vi "aft_FXP_LMS_Address_Generator.vi"(7 "filter length":i32, 10 "initialize x read address":u32, 11 "index":i32) -> (0 "x read address":u32, 1 "coefficient read address":u32, 2 "coefficient write enable":bool, 3 "coefficient write address":u32)   [LabVIEW 2017]
doc: "This VI generates addresses for reading and writing RAM."
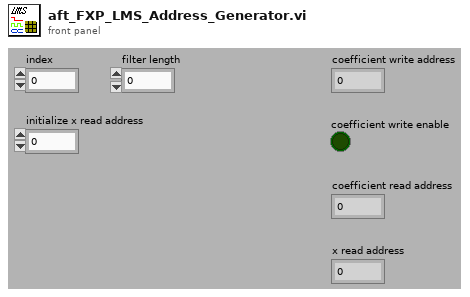
[diagram p1: front panel]
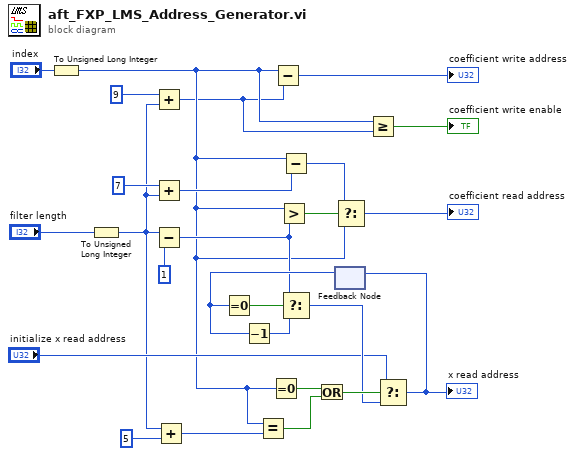
[diagram p0: block diagram]
diagram:
  n1 = To Unsigned Long Integer(number="index") -> (unsigned 32bit integer=w2:u32)
  n2 = To Unsigned Long Integer(number="filter length") -> (unsigned 32bit integer=w4:u32)
  n3 = Add(x=u32 9, y=w4) -> (x+y=w1:u32)
  n4 = Add(x=u32 7, y=w4) -> (x+y=w10:u32)
  n5 = Subtract(x=w4, y=u32 1) -> (x-y=w8:u32)
  n6 = Add(x=w4, y=u32 5) -> (x+y=w5:u32)
  n7 = Equal?(x=w2, y=w5) -> (x = y?=w22:bool)
  n8 = Equal To 0?(x=w2) -> (x = 0?=w14:bool)
  n9 = Subtract(x=w2, y=w1) -> (x-y=→"coefficient write address":u32)
  n10 = Greater?(x=w2, y=w8) -> (0:w25:bool)
  n11 = Subtract(x=w2, y=w10) -> (x-y=w24:u32)
  n12 = Or(x=w14, y=w22) -> (x .or. y?=w21:bool)
  n13 = feedback #1() -> (w16:u32)  [unwired: 1 out]
  n14 = Equal To 0?(x=w16) -> (x = 0?=w20:bool)
  n15 = Decrement(x=w16) -> (x-1=w19:u32)
  n16 = Select(t=w8, s=w20, f=w19) -> (s? t:f=w18:u32)
  n17 = Select(t=w24, s=w25, f=w2) -> (s? t:f=→"coefficient read address":u32)
  n18 = Greater Or Equal?(x=w2, y=w1) -> (x >= y?=→"coefficient write enable":bool)
  n19 = Select(t="initialize x read address", s=w21, f=w18) -> (s? t:f=w17:u32)
  "x read address" <- w17
  n20 = feedback-in #1(w17) -> ()
